vi "Database-CheckStatus.vi"(8 "error in":errorcluster, 10 "PLCcheckstatus":T2, 11 "Idx":i32) -> (0 "error out":errorcluster, 2 "PCcheckstatus":T1)   [LabVIEW 2016]
doc: "Go to DB->WriteStationValues action\nReturn boolean flag to show if data was saved to DB successfully\n\nWabco 2017 All right reserved\nAuthor: maciej.szupienko@wabco-auto.com"
uses:
  Cache/Cache.Status.Fglb.Action.ctl
  Drivers/PLC/LowLevel/PLC.DataBlock.PLCcheckstatus.ctl
  Drivers/PLC/LowLevel/PLC.DataBlock.PCcheckstatus.ctl
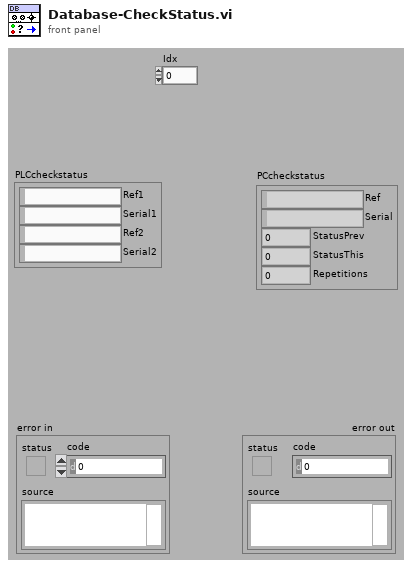
[diagram p1: front panel]
types:
  T1 = typedef "PLC.DataBlock.PCcheckstatus.ctl" = cluster{"Ref":string, "Serial":string, "StatusPrev":i8, "StatusThis":i8, "Repetitions":u8}
  T2 = typedef "PLC.DataBlock.PLCcheckstatus.ctl" = cluster{"Ref1":string, "Serial1":string, "Ref2":string, "Serial2":string}
  T3 = typedef "Cache.Status.Fglb.Action.ctl" = enum16{"init", "Changeover", "CheckStatus", "NewData", "get"}
  T4 = typedef "Database.Data.Status.ctl" = cluster{"Run":bool, "Handle":i32, "ConnTS":timestamp, "DbTime":timestamp, "DbTimeOffset":dbl, "LastVariant":string, "LastSerial":string, "LastDataTS":timestamp, "LastStatus":i32}
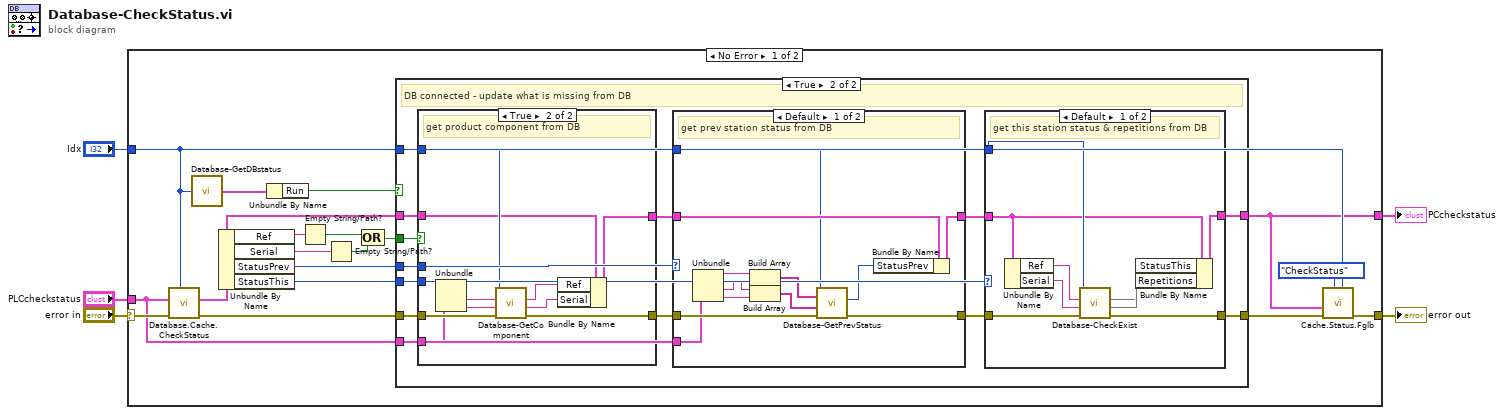
[diagram p0: block diagram]
diagram:
  n1 = case shown="No Error" "error in" {
    selector: "error in" -> [w23 w77]
    tunnel: [w9 w77] -> w4
    tunnel: "Idx" -> [w7 _]
    tunnel: [w6 _] -> w2
    tunnel: "PLCcheckstatus" -> [w11 _]
    frame No Error {
      n2 = call "Database.Cache.CheckStatus.vi"("Idx"=w7, "error in"=w23, "Data in"=w11) -> ("error out"=w18:errorcluster, "Data out"=w12:T1)  [unwired: 7 in]
      n3 = call "Database-GetDBstatus.vi"("Idx"=w7) -> ("Status"=w17:T4)
      n4 = Unbundle By Name(w12) -> ("Ref"=w22:string, "Serial"=w21:string, "StatusPrev"=w14:i8, "StatusThis"=w13:i8)
      n5 = Unbundle By Name(w17) -> ("Run"=w15:bool)
      n6 = Empty String/Path?(string/path=w22) -> (empty?=w20:bool)
      n7 = Empty String/Path?(string/path=w21) -> (empty?=w19:bool)
      n8 = Compound Arithmetic op=OR(w20, w19) -> (w16:bool)
      n9 = case shown="True" w15 {
        tunnel: w18 -> [w25 w38]
        tunnel: w16 -> [_ w37]
        tunnel: w14 -> [_ w34]
        tunnel: w13 -> [_ w33]
        tunnel: w12 -> [w24 w36]
        tunnel: w11 -> [_ w26]
        tunnel: w7 -> [_ w27]
        tunnel: [w25 w31] -> w10
        tunnel: [w24 w28] -> w6
        frame False {
          # "no connection to DB - use only information from cache"
        }
        frame True {
          # "DB connected - update what is missing from DB"
          n10 = case shown="True" w37 {
            tunnel: w38 -> [w66 w76]
            tunnel: w34 -> [_ _]
            tunnel: w33 -> [_ _]
            tunnel: w36 -> [w65 w71]
            tunnel: w26 -> [_ w74]
            tunnel: [w66 w67] -> w35
            tunnel: w27 -> [_ w75]
            tunnel: [w65 w68] -> w30
            frame False {
            }
            frame True {
              # "get product component from DB"
              n11 = Unbundle(w74) -> ("Ref2"=w73:string, "Serial2"=w72:string)  [unwired: 2 out]
              n12 = call "Database-GetComponent.vi"("error in"=w76, "Serial component"=w72, "Ref component"=w73, "Idx"=w75) -> ("error out"=w67:errorcluster, "Serial product"=w69:string, "Ref product"=w70:string)  [unwired: 5 in]
              n13 = Bundle By Name(cluster=w71, "Ref"=w70, "Serial"=w69) -> (w68:T1)
            }
          }
          n14 = case shown="Default" w34 {
            tunnel: w35 -> [w61 w64]
            tunnel: [w60 w64] -> w32
            tunnel: w30 -> [w59 w63]
            tunnel: [w62 w63] -> w29
            tunnel: w27 -> [w58 _]
            tunnel: w26 -> [w56 _]
            frame Default {
              # "get prev station status from DB"
              n15 = Unbundle(w56) -> ("Ref1"=w55:string, "Serial1"=w52:string, "Ref2"=w54:string, "Serial2"=w53:string)
              n16 = Build Array(w55, w54) -> (w51:string[])
              n17 = Build Array(w52, w53) -> (w50:string[])
              n18 = call "Database-GetPrevStatus.vi"("error in"=w61, "Serial"=w50, "Refs"=w51, "Idx"=w58) -> ("error out"=w60:errorcluster, "Status"=w57:i8)  [unwired: 6 in]
              n19 = Bundle By Name(cluster=w59, "StatusPrev"=w57) -> (w62:T1)
            }
            frame 0.. {
              # "status already found in cache"
            }
          }
          n20 = case shown="Default" w33 {
            tunnel: w32 -> [w46 w49]
            tunnel: [w41 w49] -> w31
            tunnel: w29 -> [w44 w48]
            tunnel: [w47 w48] -> w28
            tunnel: w27 -> [w45 _]
            frame Default {
              # "get this station status & repetitions from DB"
              n21 = Unbundle By Name(w44) -> ("Ref"=w43:string, "Serial"=w42:string)
              n22 = call "Database-CheckExist.vi"("error in"=w46, "Serial"=w42, "Ref"=w43, 11:w45) -> ("error out"=w41:errorcluster, 1:w40, 2:w39)  [unwired: 5 in]
              n23 = Bundle By Name(cluster=w44, "StatusThis"=w39, "Repetitions"=w40) -> (w47:T1)
            }
            frame 0.. {
              # "status already found in cache"
            }
          }
        }
      }
      n24 = call "Cache.Status.Fglb.vi"("SystemIdx"=w7, "Action (get)"=Cache.Status.Fglb.Action."CheckStatus", "error in (no error)"=w10, "CheckStatusData"=w6) -> ("error out"=w9:errorcluster)  [unwired: 6 in, 1 out]
    }
    frame Error {
    }
  }
  "error out" <- w4
  "PCcheckstatus" <- w2
